vi "Simulate Gun Software Trigger.vi"(8 "error in (no error)":errorcluster, 10 "Timeout (ms)":u32=30000) -> (0 "error out":errorcluster, 4 "Gun Trigger Time (ms)":u32=19055974)   [LabVIEW 2019]
panel:
  out "millisecond timer value out":u32=19055976
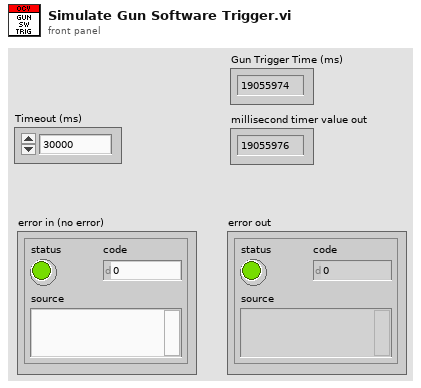
[diagram p1: front panel]
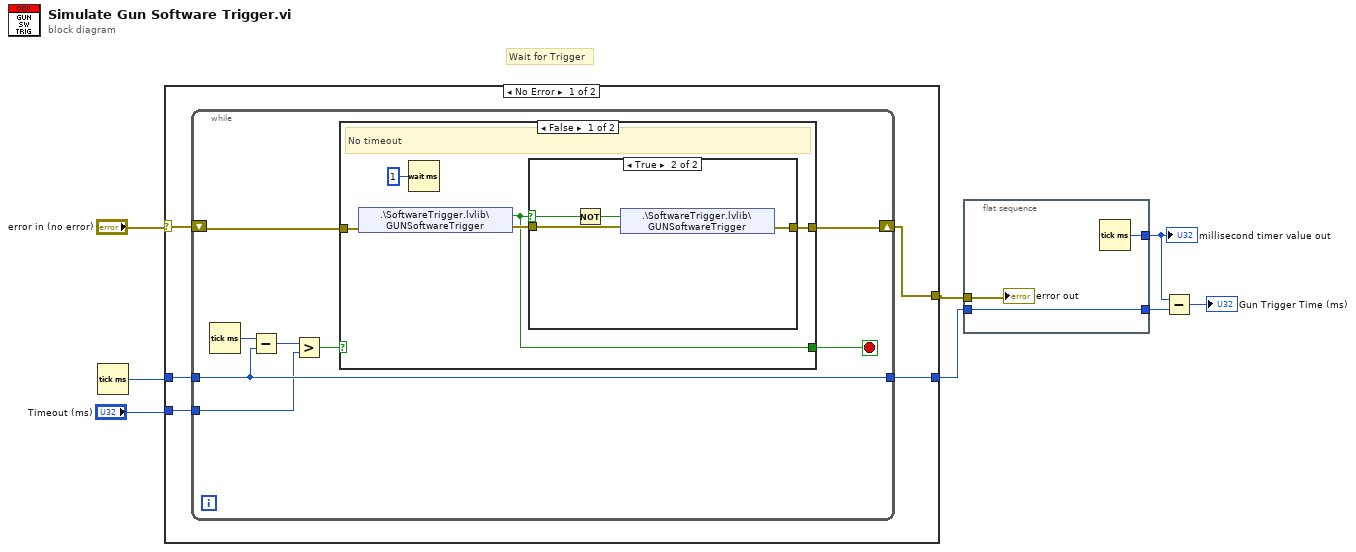
[diagram p0: block diagram]
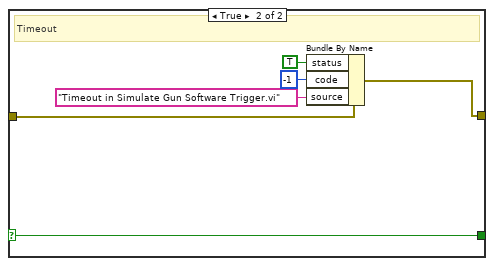
[diagram p3: hidden frame]
diagram:
  # "Wait for Trigger"
  n1 = Tick Count (ms)() -> (millisecond timer value=w4:u32)
  n2 = case shown="No Error" "error in (no error)" {
    selector: "error in (no error)" -> [w10 w39]
    tunnel: [w9 w39] -> w2
    tunnel: w4 -> [w13 w38]
    tunnel: [w12 w38] -> w1
    tunnel: "Timeout (ms)" -> [w11 _]
    frame No Error {
      n3 = while {
        shift-right: [w20] -> w9
        shift-left: w10 -> [w21]
        tunnel: w13 -> [w18]
        tunnel: [w18] -> w12
        tunnel: w11 -> [w16]
        stop <- w14 stop-if-true
        n4 = Tick Count (ms)() -> (millisecond timer value=w19:u32)
        n5 = Subtract(x=w19, y=w18) -> (x-y=w17:u32)
        n6 = Greater?(x=w17, y=w16) -> (0:w15:bool)
        n7 = case shown="False" w15 {
          selector: w15 -> [_ w37]
          tunnel: w21 -> [w25 w36]
          tunnel: [w23 w35] -> w20
          tunnel: [w22 w37] -> w14
          frame False {
            # "No timeout"
            n8 = shared-variable ".\\SoftwareTrigger.lvlib\\GUNSoftwareTrigger"(error in=w25) -> (w22:bool, error out=w24:errorcluster)
            n9 = Wait (ms)(milliseconds to wait=u32 1) -> ()  [unwired: 1 out]
            n10 = case shown="True" w22 {
              selector: w22 -> [_ w29]
              tunnel: w24 -> [w27 w31]
              tunnel: [w27 w30] -> w23
              frame False {
              }
              frame True {
                n11 = Not(x=w29) -> (.not. x?=w28:bool)
                n12 = shared-variable ".\\SoftwareTrigger.lvlib\\GUNSoftwareTrigger"(w28, error in=w31) -> (error out=w30:errorcluster)
              }
            }
          }
          frame True {
            # "Timeout"
            n13 = Bundle By Name(cluster=w36, "status"=TRUE, "code"=-1, "source"="Timeout in Simulate Gun Software Trigger.vi") -> (w35:errorcluster)
          }
        }
      }
    }
    frame Error {
    }
  }
  n14 = flat-sequence {
    tunnel: [w42] -> w6
    tunnel: w1 -> [w41]
    tunnel: [w41] -> w7
    tunnel: w2 -> [w40]
    frame #0 {
      n15 = Tick Count (ms)() -> (millisecond timer value=w42:u32)
      "error out" <- w40
    }
  }
  n16 = Subtract(x=w6, y=w7) -> (x-y=→"Gun Trigger Time (ms)":u32)
  "millisecond timer value out" <- w6
